vi "udp_incoming_filter.vi"(4 "net address":u32, 6 "port":u16, 7 "IgnoreIP":string[](array[string])=["192.168.1.11", "0.0.0.0", "127.0.0.1", "0.0.0.6"], 8 "error in (no error)":errorcluster, 9 "data includes array or string size?":bool, 10 "byte order (0:big-endian, network order)":T1(ring), 11 "received string":string) -> (0 "error out":errorcluster, 1 "data source info":cluster{"name":string, "port":u16}, 2 "Validated":bool, 3 "data string":string)   [LabVIEW 2014]
uses:
  globals/udp_validation.vi
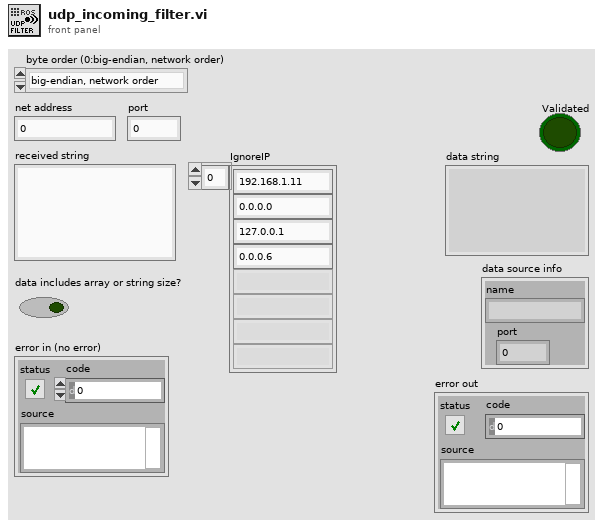
[diagram p1: front panel]
types:
  T1 = enum16{"big-endian, network order", "native, host order", "little-endian"}
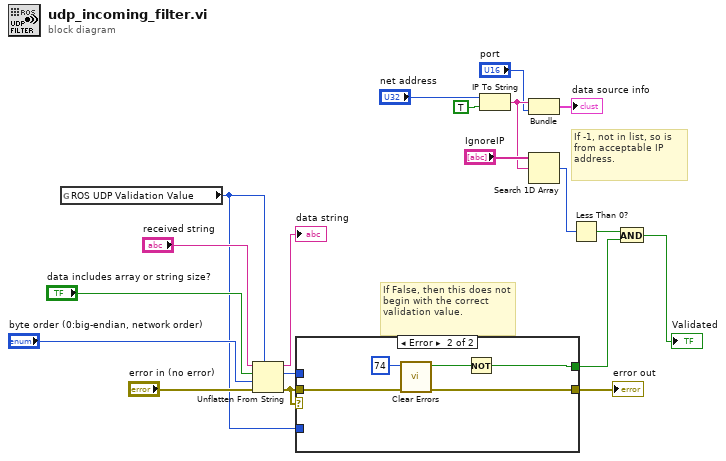
[diagram p0: block diagram]
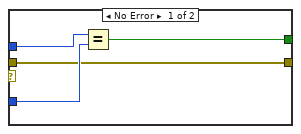
[diagram p2: hidden frame]
diagram:
  # "If False, then this does not begin with the correct validation value."
  # "If -1, not in list, so is from acceptable IP address."
  n1 = global read "udp_validation.vi" "ROS UDP Validation Value"() -> (w5:u16)
  n2 = Unflatten From String(type=w5, binary string="received string", data includes array or string size? (T)="data includes array or string size?", byte order (0:big-endian, network order)="byte order (0:big-endian, network order)", error in (no error)="error in (no error)") -> (rest of the binary string=→"data string":string, value=w6:u16, error out=w1:errorcluster)
  n3 = case shown="Error" w1 {
    tunnel: w6 -> [w23 _]
    tunnel: w5 -> [w22 _]
    tunnel: [w21 w25] -> w3
    tunnel: [w20 w27] -> w2
    tunnel: w1 -> [w20 w28]
    frame No Error {
      n4 = Equal?(x=w23, y=w22) -> (x = y?=w21:bool)
    }
    frame Error {
      n5 = call <vilib>:"Clear Errors.vi"("error in (no error)"=w28, "specific error code to clear (0: all)"=74) -> ("error out"=w27:errorcluster, "specific error cleared?"=w26:bool)  [unwired: 4 in]
      n6 = Not(x=w26) -> (.not. x?=w25:bool)
    }
  }
  "error out" <- w2
  n7 = IP To String(1:TRUE, 2:"net address") -> (0:w17:string)
  n8 = Bundle("name"=w17, "port"="port") -> (→"data source info":cluster{"name":string, "port":u16})  [unwired: 1 in]
  n9 = Search 1D Array(1D array="IgnoreIP", element=w17) -> (index of element=w16:i32)  [unwired: 1 in]
  n10 = Less Than 0?(x=w16) -> (x < 0?=w7:bool)
  n11 = And(x=w7, y=w3) -> (x .and. y?=→"Validated":bool)
